vi "Math-PDF to PMF.vi"(0 "X in":dbl[](array[numeric]), 5 "PDF":dbl[](array[numeric])) -> (4 "X out":dbl[](array[numeric]), 6 "PMF":dbl[](array[numeric]))   [LabVIEW 2020]
uses:
  <vilib>/Analysis/polynomials.llb/Unique Numbers and Multiplicity (DBL).vi
  <vilib>/Analysis/NI_AALPro.lvlib
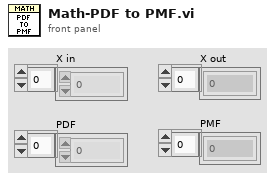
[diagram p1: front panel]
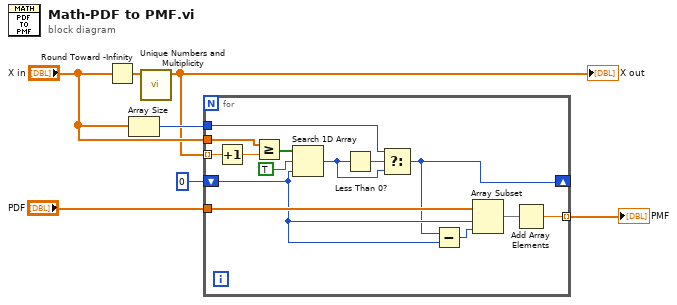
[diagram p0: block diagram]
diagram:
  n1 = Round Toward -Infinity(1:"X in") -> (0:w7:dbl[])
  n2 = Array Size(array="X in") -> (size(s)=w5:i32)
  n3 = call-poly <vilib>:"Unique Numbers and Multiplicity.vi"("Numbers"=w7) -> ("Unique Numbers"=w2:dbl[])  [unwired: 8 in, 2 out]
  "X out" <- w2
  n4 = for {
    tunnel: "X in" -> [w10]
    tunnel: w2 -> [w21] mode=indexing
    shift-right: [w12] -> _
    shift-left: 0 -> [w19]
    tunnel: "PDF" -> [w20]
    tunnel: [w16] -> w1 mode=indexing
    tunnel: w5 -> [w13]
    n5 = Increment(x=w21) -> (x+1=w11:dbl)
    n6 = Greater Or Equal?(x=w10, y=w11) -> (x >= y?=w9:bool[])
    n7 = Search 1D Array(1D array=w9, element=TRUE, start index (0)=w19) -> (index of element=w14:i32)
    n8 = Less Than 0?(x=w14) -> (x < 0?=w15:bool)
    n9 = Select(t=w13, s=w15, f=w14) -> (s? t:f=w12:i32)
    n10 = Subtract(x=w12, y=w19) -> (x-y=w18:i32)
    n11 = Array Subset(array=w20, index=w19, length=w18) -> (w17:dbl[])
    n12 = Add Array Elements(numeric array=w17) -> (sum=w16:dbl)
  }
  "PMF" <- w1
